vi "自动测试类型2统计结果.vi"   [LabVIEW 2010]
uses:
  全局量/自动测试结果.vi
  全局量/试验配置信息.vi
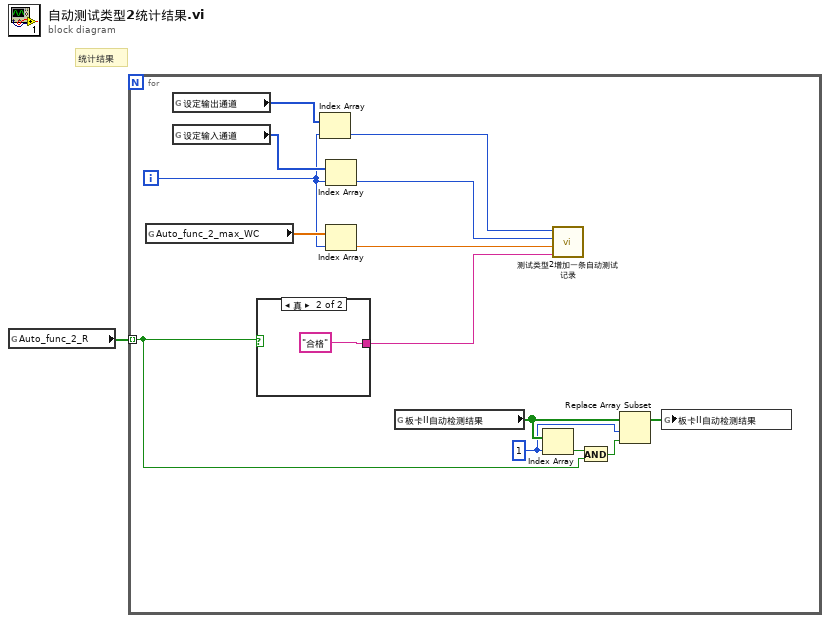
[diagram p0: block diagram]
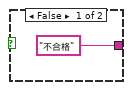
[diagram p2: hidden frame]
diagram:
  # "统计结果"
  n1 = global read "自动测试结果.vi" "Auto_func_2_R"() -> (w1:bool[])
  n2 = for {
    tunnel: w1 -> [w7] mode=indexing
    i -> [w12]
    w9 = 1 ("索引")
    n3 = global read "自动测试结果.vi" "Auto_func_2_max_WC"() -> (w15:dbl[])
    n4 = global read "试验配置信息.vi" "设定输出通道"() -> (w14:u32[])
    n5 = global read "试验配置信息.vi" "设定输入通道"() -> (w13:u32[])
    n6 = case shown="真" w7 {
      tunnel: ["不合格" "合格"] -> w2
      frame False {
      }
      frame True {
      }
    }
    n7 = Index Array(array=w14, index=w12) -> (element=w5:u32)
    n8 = Index Array(array=w13, index=w12) -> (element=w4:u32)
    n9 = Index Array(array=w15, index=w12) -> (element=w3:dbl)
    n10 = global read "试验配置信息.vi" "板卡II自动检测结果"() -> (w10:bool[])
    n11 = Index Array(array=w10, index=w9) -> (element=w8:bool)
    n12 = call "测试类型2增加一条自动测试记录.vi"("测试结果"=w2, "最大误差"=w3, "输入通道"=w4, "输出通道"=w5) -> ()  [unwired: 8 in]
    n13 = And(x=w8, y=w7) -> (x .and. y?=w6:bool)
    n14 = Replace Array Subset(array=w10, new element=w6, index=w9) -> (w11:bool[])
    n15 = global write "试验配置信息.vi" "板卡II自动检测结果"(w11) -> ()
  }
